vi "PressureChange.vi"(11 "Pressure Voltage (V)":dbl) -> (3 "Streamwise dP (kPa)":dbl)   [LabVIEW 2016]
uses:
  <vilib>/express/express arith-compare/Formula/XNode/ExpressFormulaBlockNode.xnode
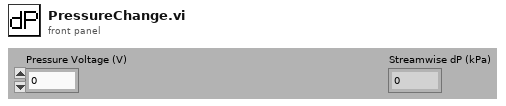
[diagram p1: front panel]
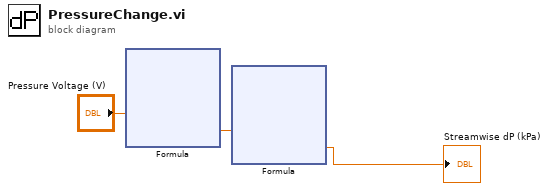
[diagram p0: block diagram]
diagram:
  n1 = xnode "Formula"("I"="Pressure Voltage (V)") -> ("Result"=w3:dbl)  [unwired: 1 in, 1 out]
  n2 = xnode "Formula"("P"=w3) -> ("Result"=→"Streamwise dP (kPa)":dbl)  [unwired: 1 in, 1 out]
